vi "Write Slew Rate.vi"(8 "error in":errorcluster, 10 "Slew Rate":dbl, 11 "Electronic Load in":refnum<class "Electronic Load.lvclass">) -> (0 "error out":errorcluster, 3 "Electronic Load out":refnum<class "Electronic Load.lvclass">)   [LabVIEW 2019, in "Electronic Load.lvlib" / "Electronic Load.lvclass"]
uses:
  Library/Electronic Load.lvclass
  C:/Users/Public/Documents/Development/builds/Instruments/Instruments.lvlibp/Library/Instruments.lvclass
  Library/Electronic Load.lvclass/Electronic Load.ctl
  builds/Instruments/Instruments.lvlibp/Private/Polymorphic/Integers/Event from DBL.vi
  builds/Instruments/Instruments.lvlibp/Accessors/Command with Logging.vi
  builds/Instruments/Instruments.lvlibp/Library/Instruments.lvclass
  builds/Instruments/Instruments.lvlibp
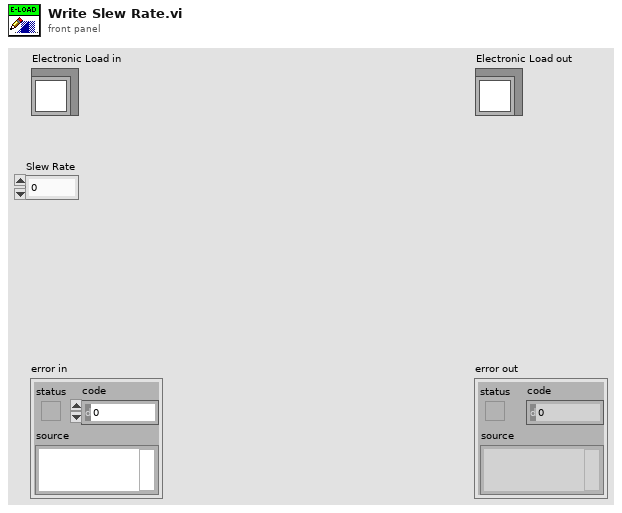
[diagram p1: front panel]
types:
  T1 = typedef "Electronic Load.lvlib/Electronic Load.lvclass/E-Load Function.ctl" = cluster{"Mode":T2, "Input Level":dbl, "Output":bool, "Slew Rate":dbl}
  T2 = typedef "Electronic Load.lvlib/Electronic Load.lvclass/E-Load Mode.ctl" = enum16{"Current", "Resistance", "Voltage"}
  T3 = cluster{"Timestamp":timestamp, "Description":string, "Data":string}
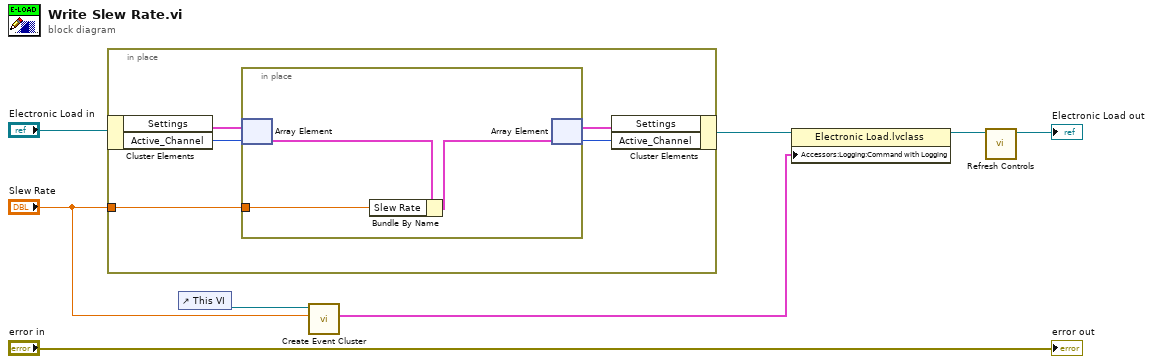
[diagram p0: block diagram]
diagram:
  n1 = in-place {
    in-place-border: "Slew Rate" -> [w9]
    n2 = in-place-cluster #1("Electronic Load in") -> ("Settings"=w13:T1[], "Active_Channel"=w12:u32)
    n3 = in-place {
      in-place-border: w9 -> [w14]
      n4 = in-place-array #2(w13, w12) -> (w16:T1)
      n5 = Bundle By Name(cluster=w16, "Slew Rate"=w14) -> (w15:T1)
      n6 = in-place-array #2(w15) -> (w11:T1[], w10:i32)
    }
    n7 = in-place-cluster #1("Settings"=w11, "Active_Channel"=w10) -> (w5:refnum<class "Electronic Load.lvclass">)
  }
  n8 = control-ref of="This VI"() -> (w6:refnum<vi>)
  n9 = call-poly "Create Event Cluster.vi"("Value"="Slew Rate", "VI Refnum"=w6) -> ("Event Data"=w4:T3)  [unwired: 9 in]
  n10 = property class="Electronic Load.lvclass"(reference=w5, "Accessors:Logging:Command with Logging"=w4) -> (reference out=w2:refnum<class "Electronic Load.lvclass">)  [unwired: 1 in, 1 out]
  n11 = call "Refresh Controls.vi"("Electronic Load in"=w2) -> ("Electronic Load out"=→"Electronic Load out":refnum<class "Electronic Load.lvclass">)  [unwired: 9 in, 1 out]
  "error out" <- "error in"
